vi "Arduino_IMU_student.vi"() -> ()   [LabVIEW 2014]
uses:
  <vilib>/Instr/_visa.llb/VISA Configure Serial Port (Instr).vi
  <vilib>/ptbypt/NI_PtbyPt.lvlib
panel:
  in  "Enable Display":bool
  out "3D Picture Control":refnum<vi>(3d-picture)
  out "Orientation (pitch, roll, yaw)":dbl[](array[numeric])
  in  "Reset":bool
  out "Magnetometer_Scale (x, y, z)":dbl[](array[numeric])
  in  "Calibrate Magnetometer?":bool
  out "Magnetometer_Offsets (x, y, z)":dbl[](array[numeric])
  out "Raw Data":string
  in  "stop":bool
  in  "Arduino Port":refnum<visa-resource-name>="COM8"
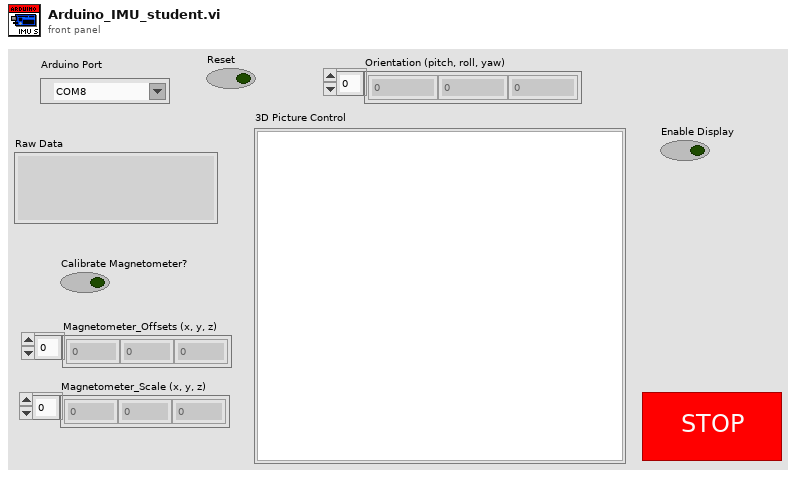
[diagram p1: front panel]
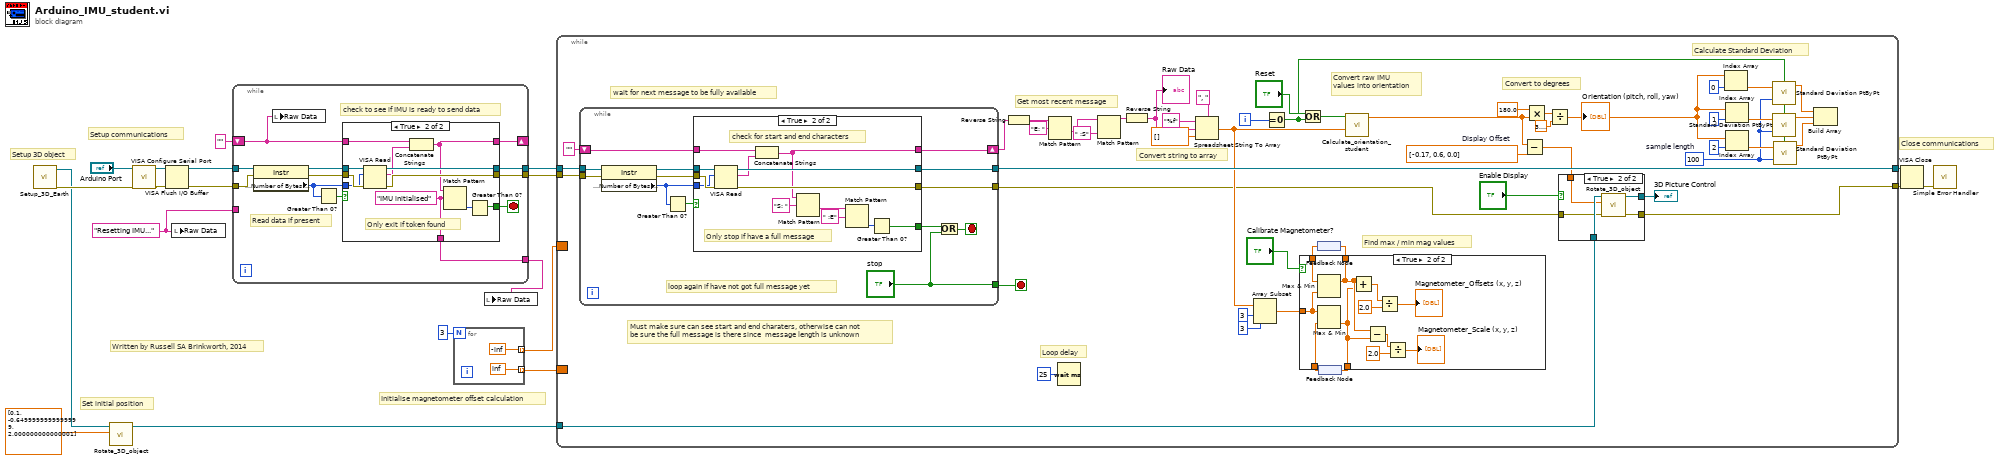
[diagram p0: block diagram]
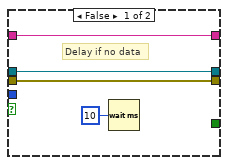
[diagram p2: hidden frame]
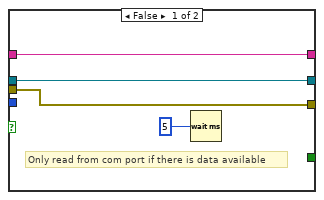
[diagram p5: hidden frame]
diagram:
  w7 = "Resetting IMU..." ("Response")
  # "Written by Russell SA Brinkworth, 2014"
  # "Set initial position"
  # "Setup 3D object"
  # "Initialise magnetometer offset calculation"
  # "Setup communications"
  # "Close communications"
  n1 = call "Setup_3D_Earth.vi"() -> ("error out"=w4:errorcluster, "SceneObject out"=w3:refnum<vi>)  [unwired: 10 in]
  n2 = call "Rotate_3D_object.vi"("Orientation (pitch, roll, yaw)"=dbl[] [0.1, -0.6499999999999999, 2.000000000000001] ("Delta_orientation (pitch, roll, yaw) 2"), "SceneObject in"=w3) -> ("SceneObject out"=w1:refnum<vi>)  [unwired: 8 in, 1 out]
  n3 = call-poly "VISA Configure Serial Port"("VISA resource name"="Arduino Port", "error in (no error)"=w4) -> ("VISA resource name out"=w13:refnum<visa-resource-name>, "error out"=w14:errorcluster)  [unwired: 7 in, 5 out]
  n4 = VISA Flush I/O Buffer(VISA resource name=w13, error in (no error)=w14) -> (VISA resource name out=w12:refnum<visa-resource-name>, error out=w10:errorcluster)  [unwired: 1 in]
  n5 = local write "Raw Data"(w7) -> ()
  n6 = while {
    tunnel: w12 -> [w31]
    tunnel: [w28] -> w11
    tunnel: w10 -> [w32]
    tunnel: [w26] -> w9
    shift-right: [w25] -> _
    shift-left: "" -> [w21]
    tunnel: [w23] -> w6
    tunnel: w7 -> [_]
    stop <- w24 stop-if-true
    # "check to see if IMU is ready to send data"
    # "Read data if present"
    n7 = property class="Instr"(reference=w31, error in=w32) -> (reference out=w29:refnum<visa-resource-name>, error out=w27:errorcluster, "Serial Settings:Number of Bytes at Serial Port"=w22:u32)
    n8 = local write "Raw Data"(w21) -> ()
    n9 = Greater Than 0?(x=w22) -> (x > 0?=w30:bool)
    n10 = case shown="True" w30 {
      tunnel: w29 -> [w36 w47]
      tunnel: [w36 w44] -> w28
      tunnel: w27 -> [w35 w46]
      tunnel: [w35 w45] -> w26
      tunnel: [w34 w41] -> w25
      tunnel: w21 -> [w34 w42]
      tunnel: [_ w39] -> w24
      tunnel: [_ w38] -> w23
      tunnel: w22 -> [_ w37]
      frame False {
        # "Delay if no data"
        n11 = Wait (ms)(milliseconds to wait=u32 10) -> ()  [unwired: 1 out]
      }
      frame True {
        w38 = "IMU initialised" ("regular expression")
        # "Only exit if token found"
        n12 = VISA Read(VISA resource name=w47, byte count=w37, error in (no error)=w46) -> (VISA resource name out=w44:refnum<visa-resource-name>, read buffer=w43:string, error out=w45:errorcluster)  [unwired: 1 out]
        n13 = Concatenate Strings(w42, w43) -> (w41:string)
        n14 = Match Pattern(string=w41, regular expression=w38) -> (offset past match=w40:i32)  [unwired: 1 in, 3 out]
        n15 = Greater Than 0?(x=w40) -> (x > 0?=w39:bool)
      }
    }
  }
  n16 = for {
    N: 3 -> [_]
    tunnel: [-inf] -> w16 mode=indexing
    tunnel: [inf] -> w5 mode=indexing
  }
  n17 = local write "Raw Data"(w6) -> ()
  n18 = while {
    tunnel: w11 -> [w95]
    tunnel: w9 -> [w99]
    tunnel: [w98] -> w19
    tunnel: [w68] -> w20
    border: w16 -> [_]
    border: w5 -> [_]
    tunnel: w1 -> [w71]
    i -> [w75]
    stop <- w96 stop-if-true
    w50 = 100  # sample length
    w64 = dbl[] [-0.17, 0.6, 0.0]  # Display Offset
    # "Calculate Standard Deviation"
    # "Loop delay"
    # "Convert raw IMU\nvalues into orientation"
    # "Convert string to array"
    # "Convert to degrees"
    # "Find max / min mag values"
    # "Must make sure can see start and end charaters, otherwise can not \nbe sure the full message is there since  message length is unknown"
    # "Get most recent message"
    # "wait for next message to be fully available"
    n19 = while {
      tunnel: w95 -> [w133]
      tunnel: w99 -> [w132]
      tunnel: [w130] -> w98
      tunnel: [w129] -> w69
      shift-right: [w128] -> w91
      shift-left: "" -> [w127]
      tunnel: ["stop"] -> w96
      stop <- w125 stop-if-true
      # "loop again if have not got full message yet"
      n20 = property class="Instr"(reference=w133, error in=w132) -> (reference out=w123:refnum<visa-resource-name>, error out=w131:errorcluster, "Serial Settings:Number of Bytes at Serial Port"=w121:u32)
      n21 = Greater Than 0?(x=w121) -> (x > 0?=w122:bool)
      n22 = case shown="True" w122 {
        tunnel: w121 -> [_ w148]
        tunnel: w123 -> [w137 w150]
        tunnel: w131 -> [w136 w149]
        tunnel: [w137 w147] -> w130
        tunnel: [w136 w146] -> w129
        tunnel: [_ w145] -> w126
        tunnel: w127 -> [w135 w141]
        tunnel: [w135 w140] -> w128
        frame False {
          # "Only read from com port if there is data available"
          n23 = Wait (ms)(milliseconds to wait=u32 5) -> ()  [unwired: 1 out]
        }
        frame True {
          # "check for start and end characters"
          # "Only stop if have a full message"
          n24 = VISA Read(VISA resource name=w150, byte count=w148, error in (no error)=w149) -> (VISA resource name out=w147:refnum<visa-resource-name>, read buffer=w142:string, error out=w146:errorcluster)  [unwired: 1 out]
          n25 = Concatenate Strings(w141, w142) -> (w140:string)
          n26 = Match Pattern(string=w140, regular expression="S: ") -> (after substring=w143:string)  [unwired: 1 in, 3 out]
          n27 = Match Pattern(string=w143, regular expression=" :E") -> (offset past match=w144:i32)  [unwired: 1 in, 3 out]
          n28 = Greater Than 0?(x=w144) -> (x > 0?=w145:bool)
        }
      }
      n29 = Or(x=w126, y="stop") -> (x .or. y?=w125:bool)
    }
    n30 = Reverse String(1:w91) -> (0:w90:string)
    n31 = Match Pattern(string=w90, regular expression="E: ") -> (after substring=w85:string)  [unwired: 1 in, 3 out]
    n32 = Wait (ms)(milliseconds to wait=u32 25) -> ()  [unwired: 1 out]
    n33 = Match Pattern(string=w85, regular expression=" :S") -> (before substring=w86:string)  [unwired: 1 in, 3 out]
    n34 = Reverse String(1:w86) -> (0:w87:string)
    "Raw Data" <- w87
    n35 = Spreadsheet String To Array(delimiter (Tab)=", ", format string="%f", spreadsheet string=w87, array type (2D Dbl)=dbl[] []) -> (array=w77:dbl[])
    n36 = Array Subset(array=w77, index=3, length=3) -> (w76:dbl[])
    n37 = Equal To 0?(x=w75) -> (x = 0?=w61:bool)
    n38 = Or(x="Reset", y=w61) -> (x .or. y?=w66:bool)
    n39 = feedback #1() -> (w82:dbl[])
    n40 = feedback #2() -> (w79:dbl[])
    n41 = case shown="True" "Calibrate Magnetometer?" {
      tunnel: w82 -> [w108 w120]
      tunnel: [w108 w114] -> w81
      tunnel: [w109 w113] -> w80
      tunnel: w76 -> [_ w118]
      tunnel: w79 -> [w109 w117]
      frame False {
      }
      frame True {
        n42 = Max & Min(x=w120, y=w118) -> (max(x,y)=w114:dbl[])  [unwired: 1 out]
        n43 = Max & Min(x=w118, y=w117) -> (min(x,y)=w113:dbl[])  [unwired: 1 out]
        n44 = Add(x=w114, y=w113) -> (x+y=w119:dbl[])
        n45 = Subtract(x=w114, y=w113) -> (x-y=w111:dbl[])
        n46 = Divide(x=w119, y=2.0) -> (x/y=→"Magnetometer_Offsets (x, y, z)":dbl[])
        n47 = Divide(x=w111, y=2.0) -> (x/y=→"Magnetometer_Scale (x, y, z)":dbl[])
      }
    }
    n48 = feedback-in #1(w81) -> ()
    n49 = feedback-in #2(w80) -> ()
    n50 = call "Calculate_orientation_student.vi"("IMU_in"=w77, "Reset"=w66) -> ("Orientation (pitch, roll, yaw)"=w63:dbl[])  [unwired: 9 in]
    n51 = Subtract(x=w63, y=w64) -> (x-y=w62:dbl[])
    n52 = Multiply(x=180.0, y=w63) -> (x*y=w73:dbl[])
    n53 = Divide(x=w73, y=3.141592653589793) -> (x/y=w60:dbl[])
    "Orientation (pitch, roll, yaw)" <- w60
    n54 = case shown="True" "Enable Display" {
      tunnel: w71 -> [w102 w107]
      tunnel: [w102 w106] -> w65
      tunnel: w69 -> [w101 w105]
      tunnel: [w101 w104] -> w68
      tunnel: w62 -> [_ w103]
      frame False {
      }
      frame True {
        n55 = call "Rotate_3D_object.vi"("error in (no error)"=w105, "Orientation (pitch, roll, yaw)"=w103, "SceneObject in"=w107) -> ("error out"=w104:errorcluster, "SceneObject out"=w106:refnum<vi>)  [unwired: 7 in]
      }
    }
    "3D Picture Control" <- w65
    n56 = Index Array(array=w60, index=0) -> (element=w56:dbl)
    n57 = Index Array(array=w60, index=1) -> (element=w55:dbl)
    n58 = Index Array(array=w60, index=2) -> (element=w54:dbl)
    n59 = call <vilib>:"Standard Deviation PtByPt.vi"("x"=w56, "sample length"=w50, "initialize"=w61) -> ("standard deviation"=w53:dbl)  [unwired: 2 out]
    n60 = call <vilib>:"Standard Deviation PtByPt.vi"("x"=w55, "sample length"=w50, "initialize"=w61) -> ("standard deviation"=w52:dbl)  [unwired: 2 out]
    n61 = call <vilib>:"Standard Deviation PtByPt.vi"("x"=w54, "sample length"=w50, "initialize"=w61) -> ("standard deviation"=w51:dbl)  [unwired: 2 out]
    n62 = Build Array(w53, w52, w51) -> ()  [unwired: 1 out]
  }
  n63 = VISA Close(VISA resource name=w19, error in (no error)=w20) -> (error out=w18:errorcluster)
  n64 = call <vilib>:"Simple Error Handler.vi"("error in (no error)"=w18) -> ()  [unwired: 1 in, 8 out]
